vi "Deadband.vi"(10 "Inputs":dbl[](array[numeric]), 11 "Deadband":dbl) -> (2 "Is Zero?":bool, 3 "Ouptuts":dbl[](array[numeric]))   [LabVIEW 2020]
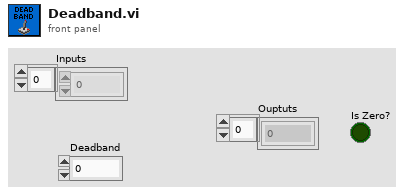
[diagram p1: front panel]
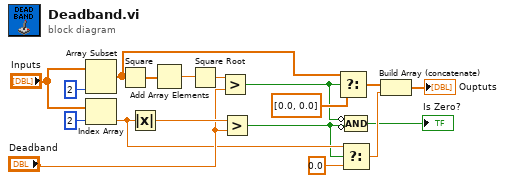
[diagram p0: block diagram]
diagram:
  n1 = Array Subset(array="Inputs", length=2) -> (w12:dbl[])  [unwired: 1 in]
  n2 = Index Array(array="Inputs", index=2) -> (element=w8:dbl)
  n3 = Square(x=w12) -> (x^2=w15:dbl[])
  n4 = Absolute Value(x=w8) -> (abs(x)=w10:dbl)
  n5 = Add Array Elements(numeric array=w15) -> (sum=w14:dbl)
  n6 = Square Root(x=w14) -> (sqrt(x)=w13:dbl)
  n7 = Greater?(x=w13, y="Deadband") -> (0:w2:bool)
  n8 = Greater?(x=w10, y="Deadband") -> (0:w1:bool)
  n9 = Select(t=w12, s=w2, f=dbl[] [0.0, 0.0]) -> (s? t:f=w6:dbl[])
  n10 = Select(t=w8, s=w1, f=0.0) -> (s? t:f=w5:dbl)
  n11 = Compound Arithmetic op=AND(invert w2, invert w1) -> (→"Is Zero?":bool)
  n12 = Build Array (concatenate)(w6, w5) -> (→"Ouptuts":dbl[])
